vi "ma_SML RT Zoom FFT (complex input).vi"(6 "reset?":bool, 7 "export time data?":bool, 8 "error in (no error)":errorcluster, 9 "zoom FFT settings":T1={"zoom settings"={"center frequency"=-inf, "zoom"=1, "trim"=1.0}, "FFT settings"={"window"=1, "window size"=-1, "FFT size"=1024, "%overlap"=0.0}} {"FFT settings"."%overlap" min=0.0 max=100.0 format="%.2f"; "FFT settings"."window" items=["Rectangle"=0, "Hanning"=1, "Hamming"=2, "Blackman-Harris"=3, "Exact Blackman"=4, "Blackman"=5, "Flat Top"=6, "4 Term B-Harris "=7, "7 Term B-Harris"=8, "Low Sidelobe"=9, "Blackman Nuttall"=11, "Triangle"=30, "Bartlett-Hanning"=31, "Bohman"=32, "Parzen"=33, "Welch"=34, "Kaiser"=60, "Dolph-Chebyshev"=61, "Gaussian"=62]; "zoom settings"."trim" min=1.0 format="%.2f"; "zoom settings"."center frequency" format="%.2f"; "zoom settings"."zoom" min=1}, 10 "fs":dbl=1024.0 format="%.2f", 11 "x":cdb[](array[numeric]) format="%.2f") -> (0 "error out":errorcluster, 1 "spectrum ready?":bool, 2 "spectral info":T3 {"window" items=["Rectangle"=0, "Hanning"=1, "Hamming"=2, "Blackman-Harris"=3, "Exact Blackman"=4, "Blackman"=5, "Flat Top"=6, "4 Term B-Harris "=7, "7 Term B-Harris"=8, "Low Sidelobe"=9, "Blackman Nuttall"=11, "Triangle"=30, "Bartlett-Hanning"=31, "Bohman"=32, "Parzen"=33, "Welch"=34, "Kaiser"=60, "Dolph-Chebyshev"=61, "Gaussian"=62]}, 3 "FFT spectrum":T4 {"spectrum" format="%.2f"; "df" format="%.2f"; "f0" format="%.2f"}, 5 "time data":T2 {"data" format="%.2f"; "dt" format="%.2f"; "t0" format="%.2f"})   [LabVIEW 2020, in "NI_MAPro.lvlib"]
uses:
  NI_MAPro.lvlib
  ma_sml_Spectrum Cluster (complex).ctl
  ma_sml_Spectral Info.ctl
  ma_sml_RT Zoom FFT Settings.ctl
  NI_AALPro.lvlib
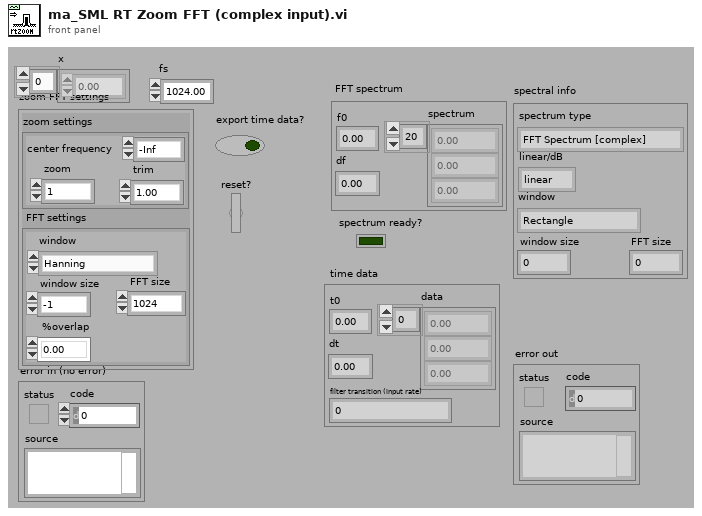
[diagram p1: front panel]
types:
  T1 = typedef "NI_MAPro.lvlib/ma_sml_RT Zoom FFT Settings.ctl" = cluster{"zoom settings":cluster{"center frequency":dbl, "zoom":i32, "trim":dbl}, "FFT settings":cluster{"window":u16, "window size":i32, "FFT size":i32, "%overlap":dbl}}
  T2 = cluster{"t0":dbl, "dt":dbl, "data":cdb[], "filter transition (input rate)":i32}
  T3 = typedef "NI_MAPro.lvlib/ma_sml_Spectral Info.ctl" = cluster{"spectrum type":enum16{"FFT Spectrum [complex]", "Amplitude [Magnitude]", "Power [Magnitude^2]", "Cross Spectrum [complex]", "Frequency Response [Complex]"}, "linear/dB":enum16{"linear", "dB"}, "window":u16, "window size":i32, "FFT size":i32}
  T4 = typedef "NI_MAPro.lvlib/ma_sml_Spectrum Cluster (complex).ctl" = cluster{"f0":dbl, "df":dbl, "spectrum":cdb[]}
  T5 = cluster{"center frequency":dbl, "zoom":i32, "trim":dbl}
  T6 = cluster{"window":u16, "window size":i32, "FFT size":i32, "%overlap":dbl}
  T7 = cluster{"zoom":i32, "stop band attenuation":enum16{"84 dB", "96 dB", "120 dB"}, "alias protect in final transition":bool, "oversampling ratio":dbl}
  T8 = cluster{"x":dbl, "dt":dbl, "Time data":cdb[], "filter transition length":i32}
  T9 = cluster{"x":dbl, "dt":dbl, "time data":cdb[], "filter transition length":i32}
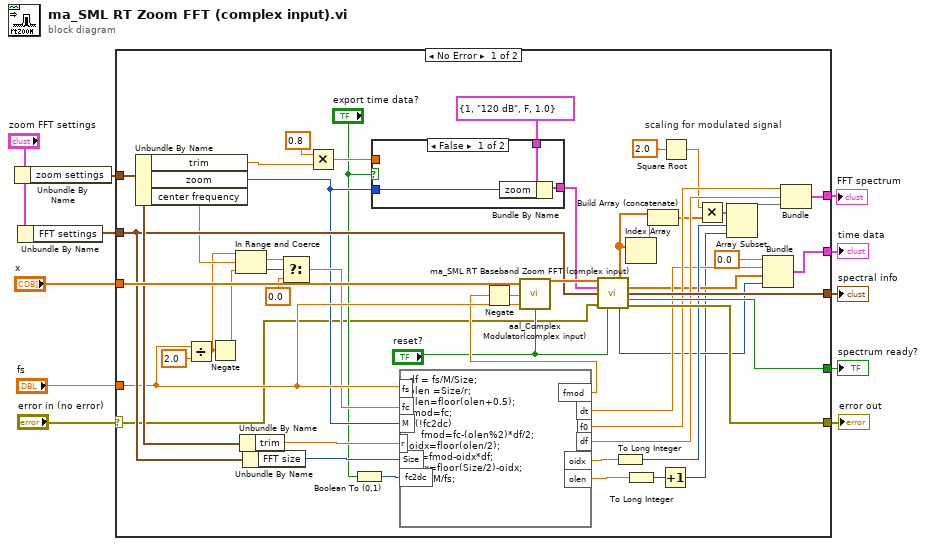
[diagram p0: block diagram]
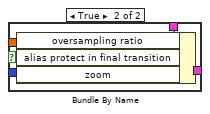
[diagram p2: hidden frame]
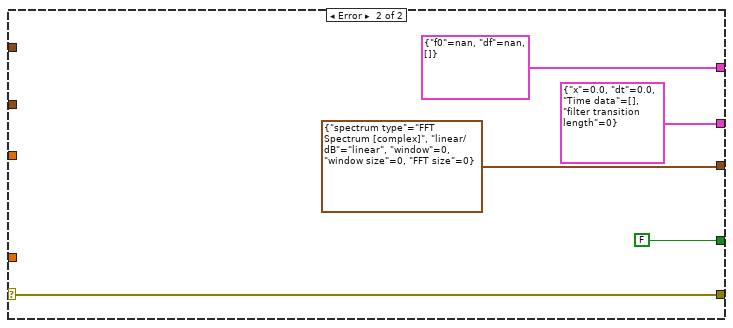
[diagram p3: hidden frame]
diagram:
  n1 = Unbundle By Name("zoom FFT settings") -> ("zoom settings"=w4:T5)
  n2 = Unbundle By Name("zoom FFT settings") -> ("FFT settings"=w3:T6)
  n3 = case shown="No Error" "error in (no error)" {
    selector: "error in (no error)" -> [w12 w71]
    tunnel: [w61 FALSE ("SpectrumReady")] -> w11
    tunnel: w4 -> [w54 _]
    tunnel: "x" -> [w60 _]
    tunnel: "fs" -> [w45 _]
    tunnel: [w50 cluster{"f0":dbl, "df":dbl, cdb[]} {"f0"=nan, "df"=nan, []}] -> w10
    tunnel: [w59 T3 {"spectrum type"=enum."FFT Spectrum [complex]", "linear/dB"=enum."linear", "window"=0, "window size"=0, "FFT size"=0} ("spectral info")] -> w8
    tunnel: [w58 w71] -> w9
    tunnel: w3 -> [w53 _]
    tunnel: [w28 T8 {"x"=0.0, "dt"=0.0, "Time data"=[], "filter transition length"=0}] -> w1
    frame No Error {
      w34 = 2.0  # scaling for modulated signal
      n4 = Unbundle By Name(w54) -> ("trim"=w23:dbl, "zoom"=w25:i32, "center frequency"=w46:dbl)
      n5 = Divide(x=w45, y=2.0) -> (x/y=w43:dbl)
      n6 = Negate(x=w43) -> (-x=w42:dbl)
      n7 = In Range and Coerce(upper limit=w43, x=w46, lower limit=w42) -> (coerced(x)=w47:dbl, In Range?=w48:bool)
      n8 = Unbundle By Name(w54) -> ("trim"=w24:dbl)
      n9 = Unbundle By Name(w53) -> ("FFT size"=w52:i32)
      n10 = Select(t=w47, s=w48, f=0.0) -> (s? t:f=w36:dbl)
      n11 = Multiply(x=0.8, y=w23) -> (x*y=w21:dbl)
      n12 = Boolean To (0,1)(Boolean="export time data?") -> (0, 1=w14:i16)
      n13 = case shown="False" "export time data?" {
        selector: "export time data?" -> [_ w67]
        tunnel: [w63 w69] -> w56
        tunnel: T7 {"zoom"=1, "stop band attenuation"=enum."120 dB", "alias protect in final transition"=FALSE, "oversampling ratio"=1.0} ("zoom settings") -> [w64 w68]
        tunnel: w25 -> [w62 w66]
        tunnel: w21 -> [_ w65]
        frame False {
          n14 = Bundle By Name(cluster=w64, "zoom"=w62) -> (w63:T7)
        }
        frame True {
          n15 = Bundle By Name(cluster=w68, "oversampling ratio"=w65, "alias protect in final transition"=w67, "zoom"=w66) -> (w69:T7)
        }
      }
      n16 = formula code="df = fs/M/Size;\nolen =Size/r;\nolen=floor(olen+0.5);\nfmod=fc;\nif(!fc2dc)\n    fmod=fc-(olen%2)*df/2;\noidx=floor(olen/2);\nf0 =fmod-oidx*df;\noidx=floor(Size/2)-oidx;\ndt = M/fs;"("fc"=w36, "M"=w25, "Size"=w52, "fs"=w45, "r"=w24, "fc2dc"=w14) -> ("f0"=w41:dbl, "df"=w49:dbl, "oidx"=w51:dbl, "olen"=w39:dbl, "dt"=w30:dbl, "fmod"=w19:dbl)
      n17 = Negate(x=w19) -> (-x=w20:dbl)
      n18 = call "aal_Complex Modulator(complex input).vi"("reset ?"="reset?", "fs"=w45, "frequency"=w20, "x"=w60) -> ("y"=w57:cdb[])
      n19 = call "ma_SML RT Baseband Zoom FFT (complex input).vi"("x [V]"=w57, "zoom settings"=w56, "FFT settings"=w53, "error in (no error)"=w12, "reset?"="reset?") -> ("FFT{X} [Vrms]"=w17:cdb[], "time data"=w29:cdb[], "spectral info"=w59:T3, "spectrum ready?"=w61:bool, "filter transition length"=w27:i32, "error out"=w58:errorcluster)  [unwired: 5 in]
      n20 = To Long Integer(number=w51) -> (32bit integer=w38:i32)
      n21 = Index Array(array=w17) -> (element=w16:cdb)  [unwired: 1 in]
      n22 = To Long Integer(number=w39) -> (32bit integer=w37:i32)
      n23 = Build Array (concatenate)(w17, w16) -> (w18:cdb[])
      n24 = Increment(x=w37) -> (x+1=w26:i32)
      n25 = Square Root(x=w34) -> (sqrt(x)=w33:dbl)
      n26 = Multiply(x=w33, y=w18) -> (x*y=w35:cdb[])
      n27 = Array Subset(array=w35, index=w38, length=w26) -> (w40:cdb[])
      n28 = Bundle("x"=0.0, "dt"=w30, "time data"=w29, "filter transition length"=w27) -> (w28:T9)  [unwired: 1 out]
      n29 = Bundle("f0"=w41, "df"=w49, w40) -> (w50:cluster{"f0":dbl, "df":dbl, cdb[]})  [unwired: 1 out]
    }
    frame Error {
    }
  }
  "spectrum ready?" <- w11
  "FFT spectrum" <- w10
  "error out" <- w9
  "spectral info" <- w8
  "time data" <- w1
